vi "数据表比对.vi"(8 "error in (no error)":errorcluster, 9 "查询元素输入":string(combo), 10 "仪器日志参数":string, 11 "table输入":string(combo)) -> (0 "error out":errorcluster, 2 "待发送第一条数据":string[](array[string]), 3 "待发送数据":string[][](table))   [LabVIEW 2016, in "数据传输系统.lvlib"]
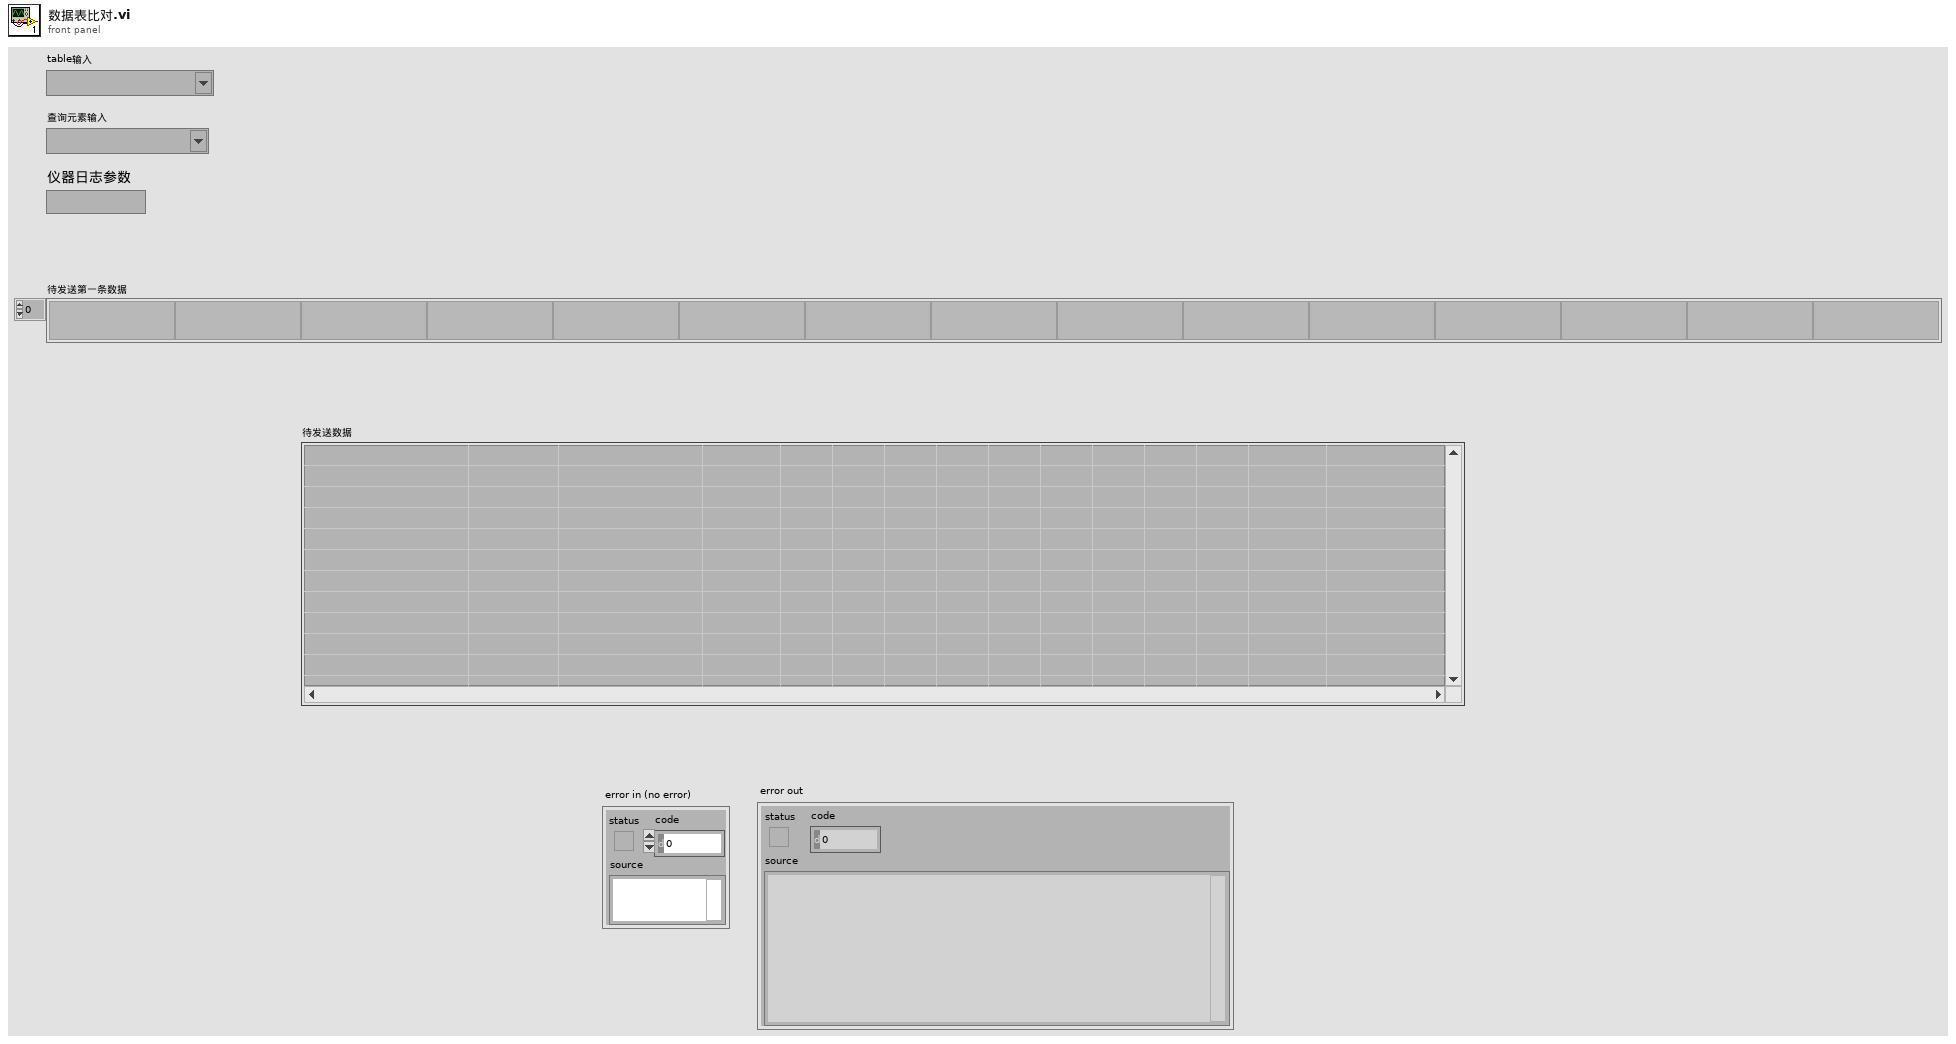
[diagram p1: front panel]
types:
  T1 = typedef "LVDateTimeRec.ctl" = cluster{"秒数的小数部分":dbl, "秒":i32, "分":i32, "时":i32, "日":i32, "月":i32, "年":i32, "天数（周）":i32, "天数（年）":i32, "DST":i32}
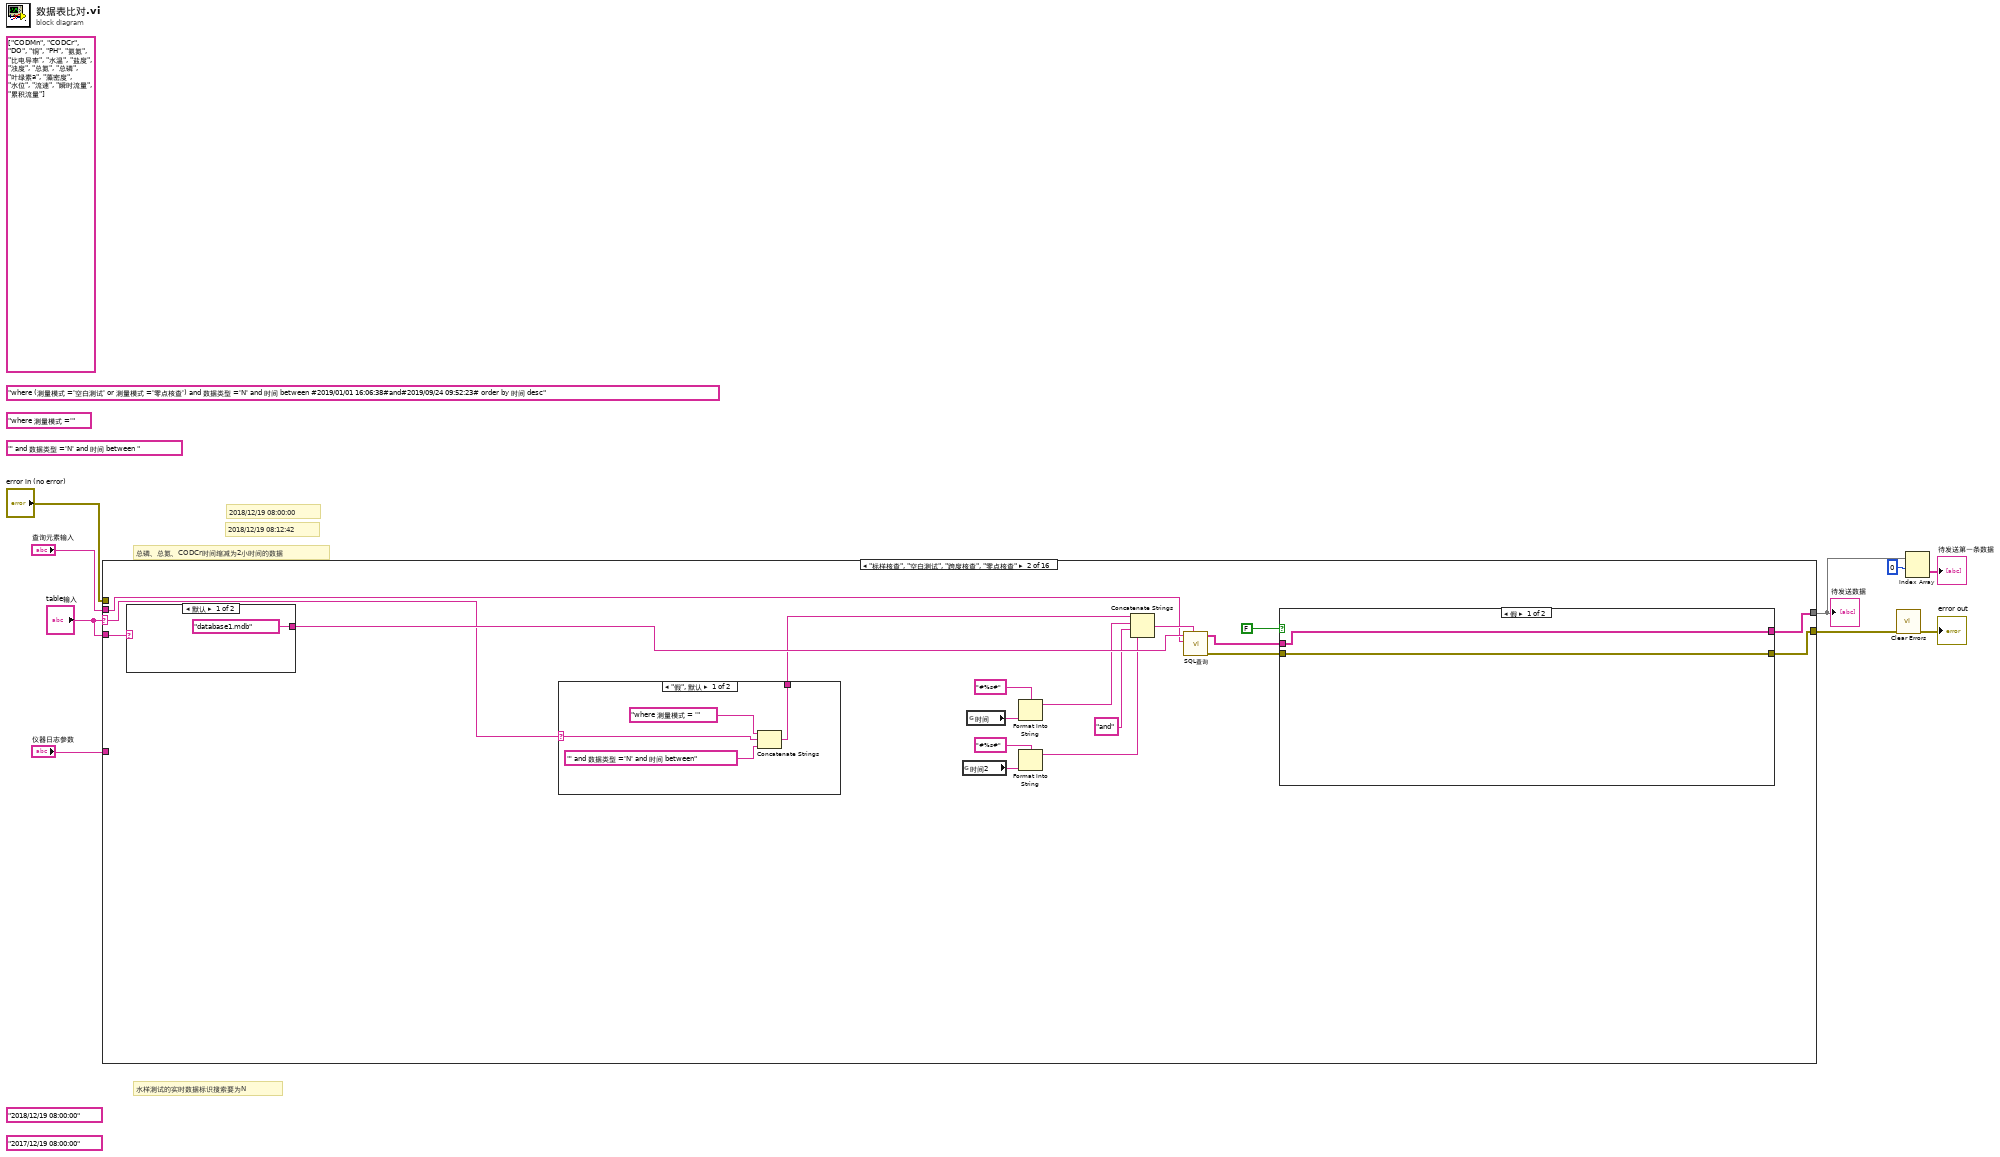
[diagram p0: block diagram]
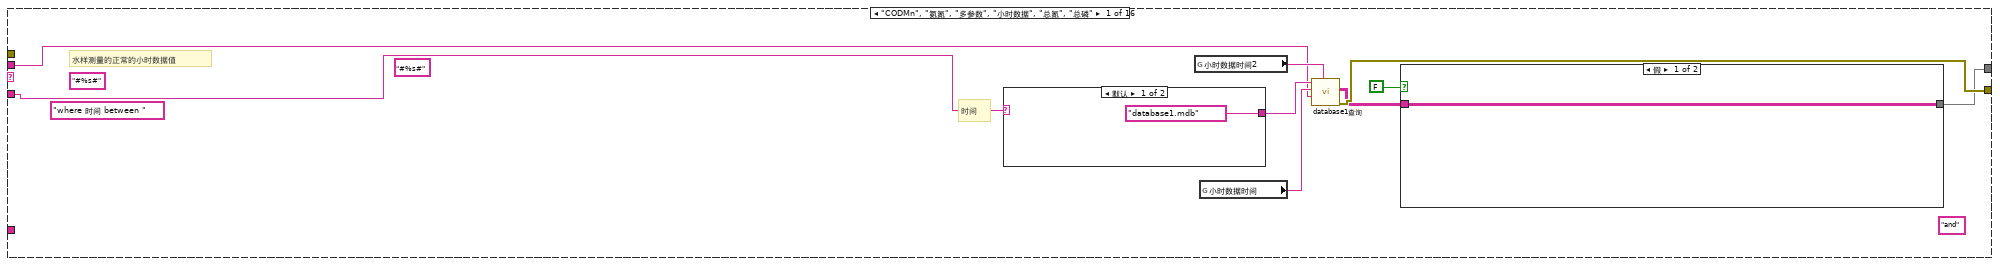
[diagram p2: hidden frame]
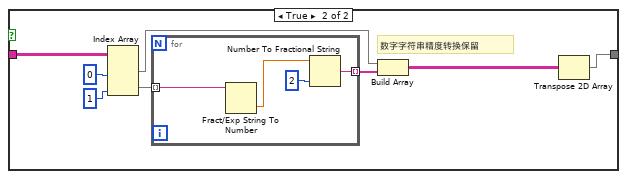
[diagram p3: hidden frame]
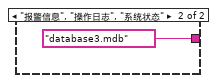
[diagram p4: hidden frame]
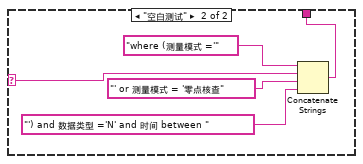
[diagram p5: hidden frame]
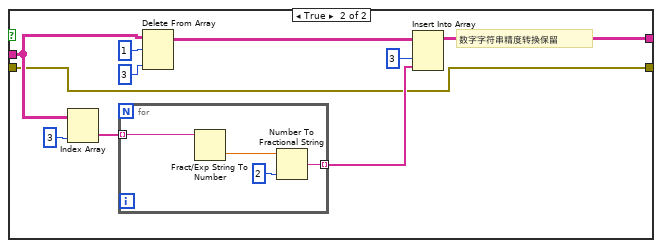
[diagram p6: hidden frame]
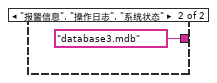
[diagram p7: hidden frame]
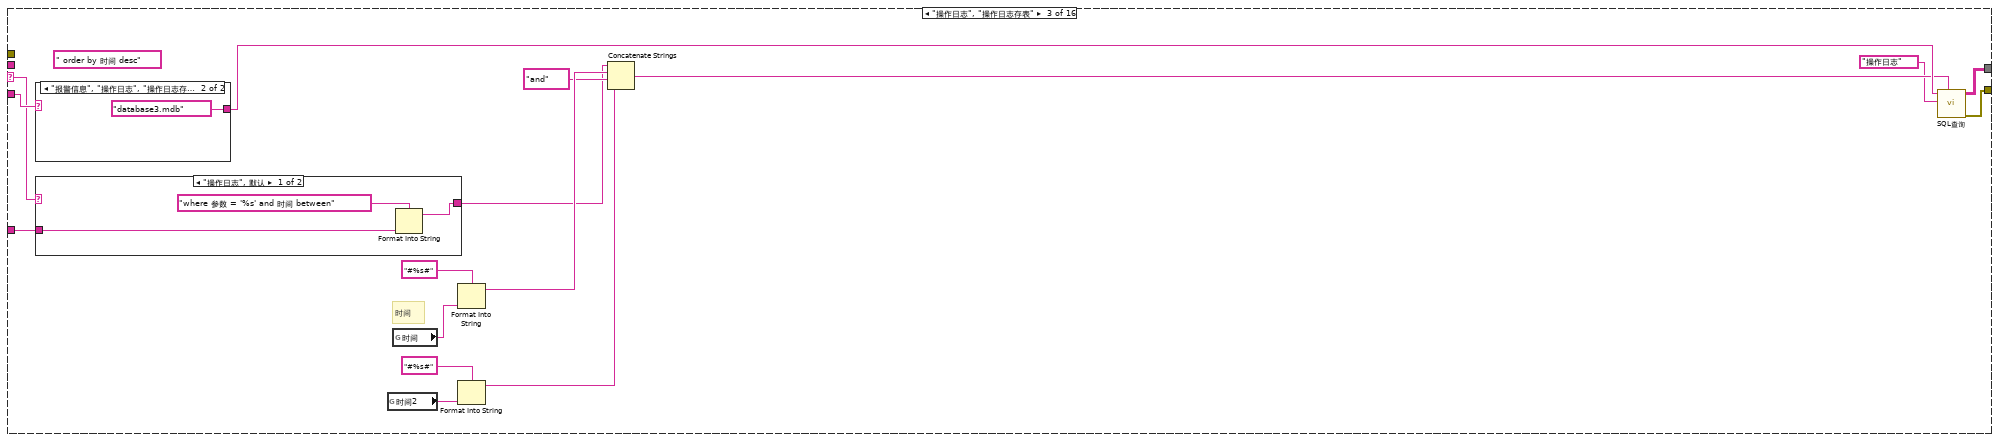
[diagram p8: hidden frame]
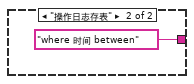
[diagram p9: hidden frame]
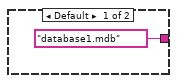
[diagram p10: hidden frame]
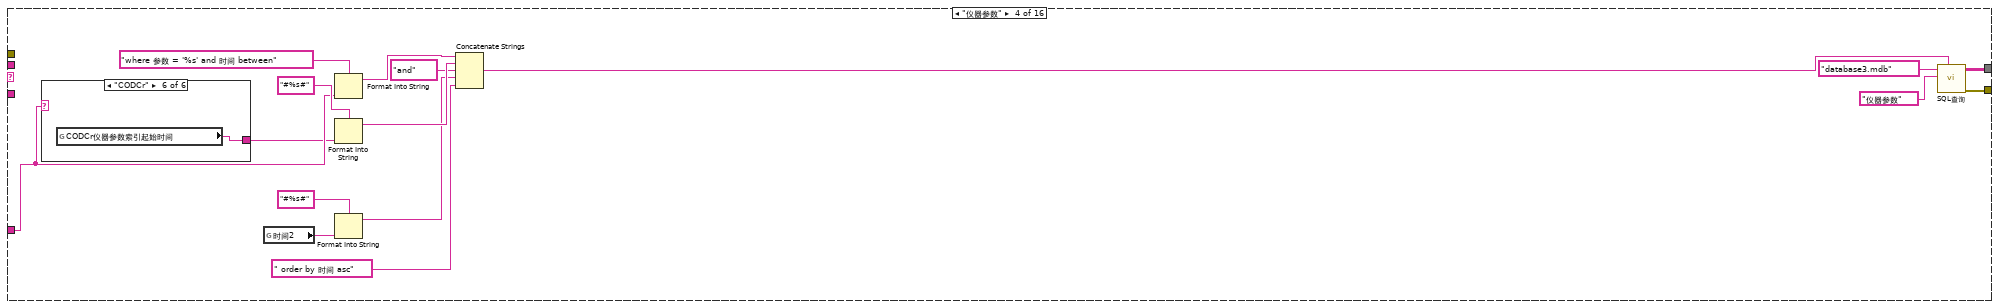
[diagram p11: hidden frame]
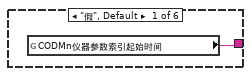
[diagram p12: hidden frame]
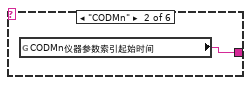
[diagram p13: hidden frame]
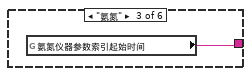
[diagram p14: hidden frame]
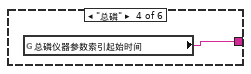
[diagram p15: hidden frame]
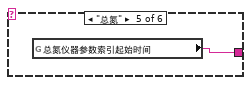
[diagram p16: hidden frame]
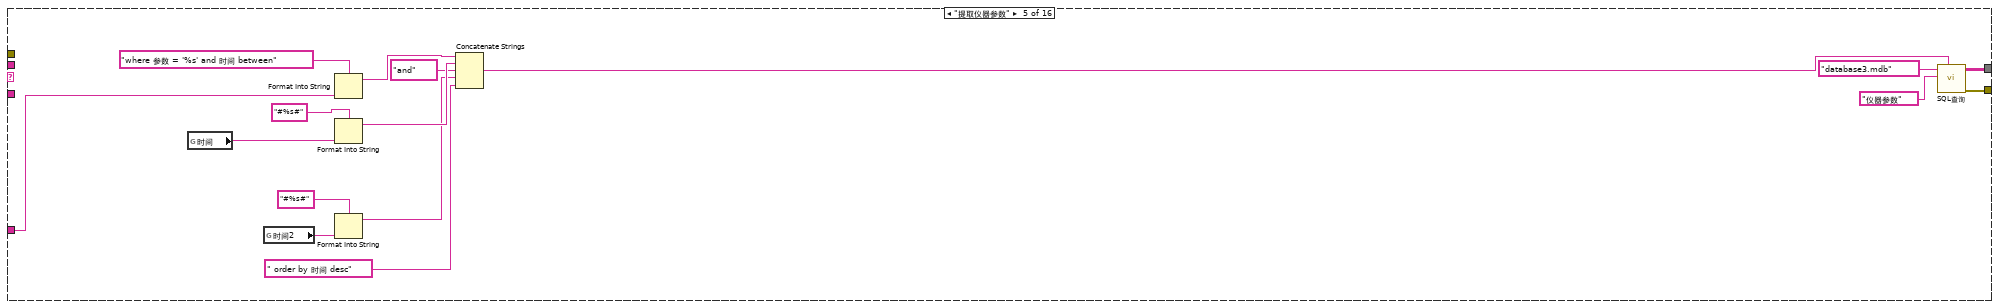
[diagram p17: hidden frame]
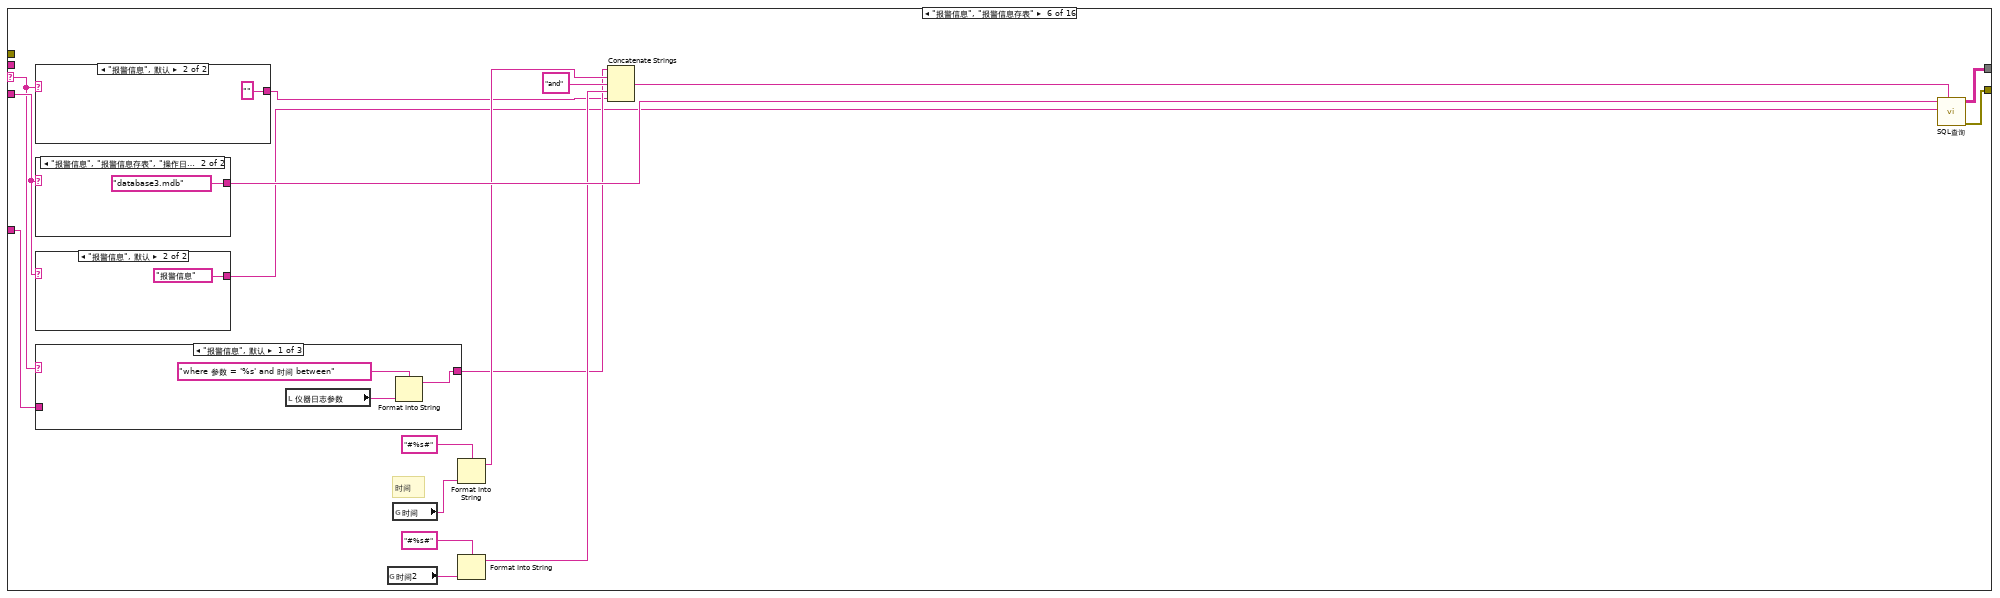
[diagram p18: hidden frame]
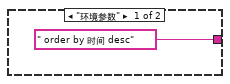
[diagram p19: hidden frame]
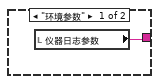
[diagram p20: hidden frame]
diagram:
  (unwired) "' and 数据类型 ='N' and 时间 between "
  (unwired) "where 测量模式 ='" ("condition")
  (unwired) "where (测量模式 ='空白测试' or 测量模式 ='零点核查') and 数据类型 ='N' and 时间 between #2019/01/01 16:06:38#and#2019/09/24 09:52:23# order by 时间 desc" ("condition")
  (unwired) string[] ["CODMn", "CODCr", "DO", "铜", "PH", "氨氮", "比电导率", "水温", "盐度", "浊度", "总氮", "总磷", "叶绿素a", "藻密度", "水位", "流速", "瞬时流量", "累积流量"] ("查询参数数组")
  (unwired) "2017/12/19 08:00:00"
  (unwired) "2018/12/19 08:00:00"
  # "水样测试的实时数据标识搜索要为N"
  # "2018/12/19 08:00:00"
  # "总磷、总氮、CODCr时间缩减为2小时间的数据"
  # "2018/12/19 08:12:42"
  n1 = case shown="\"标样核查\", \"空白测试\", \"跨度核查\", \"零点核查\"" "table输入" {
    selector: "table输入" -> [_ w35 w80 _ _ w139 _ _ _ _ _ _ _ _ _ _]
    tunnel: "error in (no error)" -> [_ _ _ _ _ _ _ w200 _ _ _ _ _ _ _ _]
    tunnel: [w16 w37 w92 w115 w137 w154 w187 w200 w215 w312 w357 w409 w461 w501 w541 w579] -> w7
    tunnel: [w12 w40 w90 w113 w135 w152 w185 w198 w218 w315 w360 w412 w464 w504 w544 w581] -> w3
    tunnel: "table输入" -> [w18 w51 w94 _ _ w142 w177 _ _ _ _ _ _ _ _ _]
    tunnel: "查询元素输入" -> [w10 w36 _ _ _ _ _ _ w201 w301 w346 w398 w454 w494 w534 w574]
    tunnel: "仪器日志参数" -> [_ _ w79 w102 w124 w140 w169 _ _ _ _ _ _ _ _ _]
    frame "CODMn", "氨氮", "多参数", "小时数据", "总氮", "总磷" {
      (unwired) "and" ("字符串")
      (unwired) "#%s#" ("初始字符串")
      (unwired) "#%s#" ("初始字符串")
      (unwired) "where 时间 between " ("condition")
      # "水样测量的正常的小时数据值"
      # "时间"
      n2 = case shown="默认" w18 {
        tunnel: ["database1.mdb" ("database") "database3.mdb" ("database")] -> w17
        frame Default {
        }
        frame "报警信息", "操作日志", "系统状态" {
        }
      }
      n3 = global read "全局 时间2.vi" "小时数据时间2"() -> (w14:string)
      n4 = global read "全局 水样时间.vi" "小时数据时间"() -> (w15:string)
      n5 = call "database1查询.vi"("时间2"=w14, "table"=w10, "时间1"=w15, "database"=w17) -> ("error out"=w16:errorcluster, "data"=w13:string[][])  [unwired: 4 in, 1 out]
      n6 = case shown="假" FALSE {
        tunnel: w13 -> [w19 w27]
        tunnel: [w19 w20] -> w12
        frame False {
        }
        frame True {
          # "数字字符串精度转换保留"
          n7 = Index Array(array=w27, index (col) #1=0 ("禁用的索引 (列)"), index (col) #2=1 ("索引 (列)")) -> (element #1=w23:string[], element #2=w24:string[])  [unwired: 2 in]
          n8 = for {
            tunnel: w24 -> [w29] mode=indexing
            tunnel: [w28] -> w22 mode=indexing
            n9 = Fract/Exp String To Number(string=w29) -> (number=w30:dbl)  [unwired: 3 in, 1 out]
            n10 = Number To Fractional String(number=w30, precision (6)=i16 2 ("精度(6)")) -> (F-format string=w28:string)  [unwired: 2 in]
          }
          n11 = Build Array(w23, w22) -> (w21:string[][])
          n12 = Transpose 2D Array(2D array=w21) -> (transposed array=w20:string[][])
        }
      }
    }
    frame "标样核查", "空白测试", "跨度核查", "零点核查" {
      n13 = case shown="默认" w51 {
        tunnel: ["database1.mdb" ("database") "database3.mdb" ("database")] -> w50
        frame Default {
        }
        frame "报警信息", "操作日志", "系统状态" {
        }
      }
      n14 = case shown="\"假\", 默认" w35 {
        selector: w35 -> [w54 w57]
        tunnel: [w52 w56] -> w34
        frame "假", Default {
          n15 = Concatenate Strings("where 测量模式 = '" ("condition"), w54, "' and 数据类型 ='N' and 时间 between" ("字符串")) -> (w52:string)
        }
        frame "空白测试" {
          n16 = Concatenate Strings("where (测量模式 ='" ("condition"), w57, "' or 测量模式 = '零点核查", "') and 数据类型 ='N' and 时间 between ") -> (w56:string)
        }
      }
      n17 = global read "全局 时间2.vi" "时间2"() -> (w42:string)
      n18 = global read "全局 水样时间.vi" "时间"() -> (w43:string)
      n19 = Format Into String(format string="#%s#" ("初始字符串"), w43) -> (resulting string=w49:string)  [unwired: 2 in, 1 out]
      n20 = Format Into String(format string="#%s#" ("初始字符串"), w42) -> (resulting string=w45:string)  [unwired: 2 in, 1 out]
      n21 = Concatenate Strings(w34, w49, "and" ("字符串"), w45) -> (w44:string)
      n22 = call "SQL查询.vi"("condition"=w44, "table输入"=w36, "database"=w50) -> ("error out"=w38:errorcluster, "data"=w41:string[][])  [unwired: 7 in]
      n23 = case shown="假" FALSE {
        tunnel: w41 -> [w62 w65]
        tunnel: [w62 w64] -> w40
        tunnel: [w61 w63] -> w37
        tunnel: w38 -> [w61 w63]
        frame False {
        }
        frame True {
          # "数字字符串精度转换保留"
          n24 = Index Array(array=w65, index (col)=3 ("禁用的索引 (列)")) -> (element=w71:string[])  [unwired: 1 in]
          n25 = for {
            tunnel: w71 -> [w74] mode=indexing
            tunnel: [w73] -> w67 mode=indexing
            n26 = Fract/Exp String To Number(string=w74) -> (number=w75:dbl)  [unwired: 3 in, 1 out]
            n27 = Number To Fractional String(number=w75, precision (6)=i16 2 ("精度(6)")) -> (F-format string=w73:string)  [unwired: 2 in]
          }
          n28 = Delete From Array(array=w65, length=1 ("长度"), index (col)=3 ("禁用的索引 (列)")) -> (array with subset deleted=w68:string[][])  [unwired: 1 in, 1 out]
          n29 = Insert Into Array(array=w68, index (col)=3 ("禁用的索引 (列)"), new element=w67) -> (w64:string[][])  [unwired: 1 in]
        }
      }
    }
    frame "操作日志", "操作日志存表" {
      (unwired) " order by 时间 desc" ("字符串")
      # "时间"
      n30 = case shown="\"报警信息\", \"操作日志\", \"操作日志存表\", \"系统状态\"" w94 {
        tunnel: ["database1.mdb" ("database") "database3.mdb" ("database")] -> w93
        frame Default {
        }
        frame "报警信息", "操作日志", "操作日志存表", "系统状态" {
        }
      }
      n31 = case shown="\"操作日志\", 默认" w80 {
        tunnel: [w96 "where 时间 between" ("condition")] -> w82
        tunnel: w79 -> [w95 _]
        frame "操作日志", Default {
          n32 = Format Into String(format string="where 参数 = '%s' and 时间 between" ("condition"), w95) -> (resulting string=w96:string)  [unwired: 2 in, 1 out]
        }
        frame "操作日志存表" {
        }
      }
      n33 = global read "全局 时间2.vi" "时间2"() -> (w83:string)
      n34 = global read "全局 水样时间.vi" "时间"() -> (w84:string)
      n35 = Format Into String(format string="#%s#" ("初始字符串"), w84) -> (resulting string=w89:string)  [unwired: 2 in, 1 out]
      n36 = Format Into String(format string="#%s#" ("初始字符串"), w83) -> (resulting string=w85:string)  [unwired: 2 in, 1 out]
      n37 = Concatenate Strings(w82, w89, "and" ("字符串"), w85) -> (w91:string)
      n38 = call "SQL查询.vi"("condition"=w91, "table输入"="操作日志", "database"=w93) -> ("error out"=w92:errorcluster, "data"=w90:string[][])  [unwired: 7 in]
    }
    frame "仪器参数" {
      n39 = case shown="\"CODCr\"" w102 {
        tunnel: [w117 w118 w119 w120 w121 w122] -> w101
        frame "假", Default {
          n40 = global read "全局 时间2.vi" "CODMn仪器参数索引起始时间"() -> (w117:string)
        }
        frame "CODMn" {
          n41 = global read "全局 时间2.vi" "CODMn仪器参数索引起始时间"() -> (w118:string)
        }
        frame "氨氮" {
          n42 = global read "全局 时间2.vi" "氨氮仪器参数索引起始时间"() -> (w119:string)
        }
        frame "总磷" {
          n43 = global read "全局 时间2.vi" "总磷仪器参数索引起始时间"() -> (w120:string)
        }
        frame "总氮" {
          n44 = global read "全局 时间2.vi" "总氮仪器参数索引起始时间"() -> (w121:string)
        }
        frame "CODCr" {
          n45 = global read "全局 时间2.vi" "CODCr仪器参数索引起始时间"() -> (w122:string)
        }
      }
      n46 = global read "全局 时间2.vi" "时间2"() -> (w107:string)
      n47 = Format Into String(format string="where 参数 = '%s' and 时间 between" ("condition"), w102) -> (resulting string=w106:string)  [unwired: 2 in, 1 out]
      n48 = Format Into String(format string="#%s#" ("初始字符串"), w101) -> (resulting string=w112:string)  [unwired: 2 in, 1 out]
      n49 = Format Into String(format string="#%s#" ("初始字符串"), w107) -> (resulting string=w108:string)  [unwired: 2 in, 1 out]
      n50 = Concatenate Strings(w106, w112, "and" ("字符串"), w108, " order by 时间 asc" ("字符串")) -> (w114:string)
      n51 = call "SQL查询.vi"("condition"=w114, "table输入"="仪器参数", "database"="database3.mdb") -> ("error out"=w115:errorcluster, "data"=w113:string[][])  [unwired: 7 in]
    }
    frame "提取仪器参数" {
      n52 = global read "全局 水样时间.vi" "时间"() -> (w123:string)
      n53 = global read "全局 时间2.vi" "时间2"() -> (w129:string)
      n54 = Format Into String(format string="where 参数 = '%s' and 时间 between" ("condition"), w124) -> (resulting string=w128:string)  [unwired: 2 in, 1 out]
      n55 = Format Into String(format string="#%s#" ("初始字符串"), w123) -> (resulting string=w134:string)  [unwired: 2 in, 1 out]
      n56 = Format Into String(format string="#%s#" ("初始字符串"), w129) -> (resulting string=w130:string)  [unwired: 2 in, 1 out]
      n57 = Concatenate Strings(w128, w134, "and" ("字符串"), w130, " order by 时间 desc" ("字符串")) -> (w136:string)
      n58 = call "SQL查询.vi"("condition"=w136, "table输入"="仪器参数", "database"="database3.mdb") -> ("error out"=w137:errorcluster, "data"=w135:string[][])  [unwired: 7 in]
    }
    frame "报警信息", "报警信息存表" {
      # "时间"
      n59 = case shown="\"报警信息\", 默认" w139 {
        tunnel: [" order by 时间 desc" ("字符串") "" ("仪器日志参数")] -> w141
        frame "环境参数" {
        }
        frame "报警信息", Default {
        }
      }
      n60 = case shown="\"报警信息\", \"报警信息存表\", \"操作日志\", \"系统状态\"" w142 {
        tunnel: ["database1.mdb" ("database") "database3.mdb" ("database")] -> w155
        frame Default {
        }
        frame "报警信息", "报警信息存表", "操作日志", "系统状态" {
        }
      }
      n61 = case shown="\"报警信息\", 默认" w142 {
        tunnel: [w158 "报警信息" ("table输入")] -> w143
        frame "环境参数" {
          n62 = local read "仪器日志参数"() -> (w158:string)
        }
        frame "报警信息", Default {
        }
      }
      n63 = case shown="\"报警信息\", 默认" w139 {
        tunnel: [w161 w164 "where 时间 between" ("condition")] -> w144
        tunnel: w140 -> [_ w163 _]
        frame "报警信息", Default {
          n64 = local read "仪器日志参数"() -> (w160:string)
          n65 = Format Into String(format string="where 参数 = '%s' and 时间 between" ("condition"), w160) -> (resulting string=w161:string)  [unwired: 2 in, 1 out]
        }
        frame "环境参数" {
          n66 = Format Into String(format string="where 参数 = '%s' and 时间 between" ("condition"), w163) -> (resulting string=w164:string)  [unwired: 2 in, 1 out]
        }
        frame "报警信息存表" {
        }
      }
      n67 = global read "全局 时间2.vi" "时间2"() -> (w145:string)
      n68 = global read "全局 水样时间.vi" "时间"() -> (w146:string)
      n69 = Format Into String(format string="#%s#" ("初始字符串"), w146) -> (resulting string=w151:string)  [unwired: 2 in, 1 out]
      n70 = Format Into String(format string="#%s#" ("初始字符串"), w145) -> (resulting string=w147:string)  [unwired: 2 in, 1 out]
      n71 = Concatenate Strings(w144, w151, "and" ("字符串"), w147, w141) -> (w153:string)
      n72 = call "SQL查询.vi"("condition"=w153, "table输入"=w143, "database"=w155) -> ("error out"=w154:errorcluster, "data"=w152:string[][])  [unwired: 7 in]
    }
    frame "环境参数" {
      n73 = case shown="默认" w177 {
        tunnel: ["database1.mdb" ("database") "database3.mdb" ("database")] -> w188
        frame Default {
        }
        frame "报警信息", "报警信息存表", "操作日志", "系统状态" {
        }
      }
      n74 = case shown="\"环境参数\"" w169 {
        tunnel: [w192 "where 时间 between" ("condition") "where 时间 between" ("condition")] -> w179
        frame "报警信息", Default {
          n75 = local read "仪器日志参数"() -> (w191:string)
          n76 = Format Into String(format string="where 参数 = '%s' and 时间 between" ("condition"), w191) -> (resulting string=w192:string)  [unwired: 2 in, 1 out]
        }
        frame "环境参数" {
        }
        frame "报警信息存表" {
        }
      }
      n77 = case shown="\"环境参数\"" w177 {
        tunnel: [w189 "报警信息" ("table输入")] -> w178
        tunnel: w169 -> [w189 _]
        frame "环境参数" {
        }
        frame "报警信息", Default {
        }
      }
      n78 = Get Date/Time In Seconds() -> (seconds since 1Jan1904=w174:timestamp)
      n79 = Seconds To Date/Time(time stamp (now)=w174) -> (date time rec=w171:T1)  [unwired: 1 in]
      n80 = Date/Time To Seconds(2:w171) -> (0:w173:timestamp)  [unwired: 1 in]
      n81 = Format Date/Time String(time format string (%c)="%Y/%m/%d %H:%M:%S" ("时间格式字符串(%c)"), seconds (now)=w173) -> (date/time string=w170:string)  [unwired: 1 in]
      n82 = Format Into String(format string="#%s#" ("初始字符串"), w170) -> (resulting string=w180:string)  [unwired: 2 in, 1 out]
      n83 = Format Into String(format string="#%s#" ("初始字符串"), "1904/01/01 00:00:00") -> (resulting string=w184:string)  [unwired: 2 in, 1 out]
      n84 = Concatenate Strings(w179, w184, "and" ("字符串"), w180, " order by 时间 desc" ("字符串")) -> (w186:string)
      n85 = call "SQL查询.vi"("condition"=w186, "table输入"=w178, "database"=w188) -> ("error out"=w187:errorcluster, "data"=w185:string[][])  [unwired: 7 in]
    }
    frame Default {
      # "时间格式转换"
      n86 = local read "待发送数据"() -> (w199:string[][])
      n87 = call "数组时间戳格式化(子VI).vi"("待发送数据输入"=w199) -> ("待发送数据输出"=w198:string[][])  [unwired: 10 in]
    }
    frame "实时数据" {
      (unwired) " order by 时间 desc" ("字符串")
      # "空白测试or零点核查要加括号"
      # "上传本地时间点的实时数据"
      # "上传质控数据（空白测试，跨度核查，核查数据，平行样数据）"
      n88 = global read "全局 实时数据参数.vi" "实时数据参数"() -> (w211:string)
      n89 = case shown="\"空白测试\"" w211 {
        tunnel: [w235 w257 w268 w274] -> w212
        tunnel: w211 -> [w231 w256 _ w270]
        tunnel: [w234 w252 w264 w269] -> w206
        tunnel: w201 -> [_ w251 _ _]
        frame "水样测试" {
          n90 = Get Date/Time In Seconds() -> (seconds since 1Jan1904=w243:timestamp)
          n91 = Format Date/Time String(time format string (%c)="%Y%m%d%H%M%S%3u" ("时间格式字符串(%c)"), seconds (now)=w243) -> (date/time string=w241:string)  [unwired: 1 in]
          n92 = local read "查询元素输入"() -> (w236:string)
          n93 = Concatenate Strings("where 测量模式 ='" ("condition"), w231, "' and 数据类型 ='N' and 时间 between ") -> (w234:string)
          n94 = Replace Substring(2:8 ("长度（子字符串长度）"), 3:10 ("偏移量(0)"), 4:"0000" ("子字符串(\"\")"), 5:w241) -> (1:w237:string)  [unwired: 1 out]
          n95 = case shown="\"CODCr\", \"CODMn\", \"累积流量\", \"总氮\", \"总磷\"" w236 {
            tunnel: w237 -> [w245 w248 _]
            tunnel: [w244 w249 w250] -> w235
            frame Default {
              n96 = Search and Replace String(input string=w245, search string="." ("搜索字符串")) -> (result string=w246:string)  [unwired: 6 in, 3 out]
              n97 = call "格式时间字符串.vi"("字符串"=w246) -> ("连接的字符串"=w244:string)  [unwired: 10 in]
            }
            frame "CODCr", "CODMn", "累积流量", "总氮", "总磷" {
              n98 = call "实时数据查询用2小时间的数据.vi"("字符串"=w248) -> ("连接的字符串"=w249:string)  [unwired: 10 in]
            }
            frame "CODCr加标回收率", "CODMn加标回收率", "氨氮加标回收率", "总氮加标回收率", "总磷加标回收率" {
              n99 = global read "全局 时间2.vi" "加标回收索引起始时间"() -> (w250:string)
            }
          }
        }
        frame "空白测试" {
          n100 = case shown="\"氨氮\"" w251 {
            tunnel: [w258 w259 w260 w261 w262 w263] -> w257
            frame "CODMn" {
              n101 = global read "全局 时间2.vi" "CODMn零点核查索引起始时间"() -> (w258:string)
            }
            frame "CODCr" {
              n102 = global read "全局 时间2.vi" "CODCr零点核查索引起始时间"() -> (w259:string)
            }
            frame "氨氮" {
              n103 = global read "全局 时间2.vi" "氨氮零点核查索引起始时间"() -> (w260:string)
            }
            frame "总磷" {
              n104 = global read "全局 时间2.vi" "总磷零点核查索引起始时间"() -> (w261:string)
            }
            frame "总氮" {
              n105 = global read "全局 时间2.vi" "总氮零点核查索引起始时间"() -> (w262:string)
            }
            frame "", Default {
              n106 = global read "全局 时间2.vi" "零点核查索引起始时间"() -> (w263:string)
            }
          }
          n107 = Concatenate Strings("where (测量模式 ='" ("condition"), w256, "' or 测量模式 = '零点核查", "') and 数据类型 ='N' and 时间 between ") -> (w252:string)
        }
        frame "核查数据" {
          n108 = global read "全局 时间2.vi" "标样核查索引起始时间"() -> (w268:string)
          n109 = Concatenate Strings("where 测量模式 ='" ("condition"), "标样核查" ("实时数据参数"), "' and 数据类型 ='N' and 时间 between ") -> (w264:string)
        }
        frame "跨度核查", Default {
          n110 = local read "查询元素输入"() -> (w273:string)
          n111 = Concatenate Strings("where 测量模式 ='" ("condition"), w270, "' and 数据类型 ='N' and 时间 between ") -> (w269:string)
          n112 = case shown="\"氨氮\"" w273 {
            tunnel: [w275 w276 w277 w278 w279 w280] -> w274
            frame "CODMn" {
              n113 = global read "全局 时间2.vi" "CODMn跨度核查索引起始时间"() -> (w275:string)
            }
            frame "CODCr" {
              n114 = global read "全局 时间2.vi" "CODCr跨度核查索引起始时间"() -> (w276:string)
            }
            frame "氨氮" {
              n115 = global read "全局 时间2.vi" "氨氮跨度核查索引起始时间"() -> (w277:string)
            }
            frame "总磷" {
              n116 = global read "全局 时间2.vi" "总磷跨度核查索引起始时间"() -> (w278:string)
            }
            frame "总氮" {
              n117 = global read "全局 时间2.vi" "总氮跨度核查索引起始时间"() -> (w279:string)
            }
            frame "", Default {
              n118 = global read "全局 时间2.vi" "跨度核查索引起始时间"() -> (w280:string)
            }
          }
        }
      }
      n119 = global read "断电保存全局.vi" "数据组合发送"() -> (w203:bool)
      n120 = Get Date/Time In Seconds() -> (seconds since 1Jan1904=w210:timestamp)
      n121 = Seconds To Date/Time(time stamp (now)=w210) -> (date time rec=w205:T1)  [unwired: 1 in]
      n122 = case shown="假" w203 {
        tunnel: w205 -> [w225 w228]
        tunnel: [w225 w226] -> w204
        frame False {
        }
        frame True {
          n123 = Unbundle By Name(w228) -> ("时"=w230:i32)
          n124 = Subtract(x=w230, y=2) -> (x-y=w227:i32)
          n125 = Bundle By Name(cluster=w228, "时"=w227) -> (w226:T1)
        }
      }
      n126 = Date/Time To Seconds(2:w204) -> (0:w209:timestamp)  [unwired: 1 in]
      n127 = Format Date/Time String(time format string (%c)="%Y/%m/%d %H:%M:%S" ("时间格式字符串(%c)"), seconds (now)=w209) -> (date/time string=w207:string)  [unwired: 1 in]
      n128 = Format Into String(format string="#%s#" ("初始字符串"), w212) -> (resulting string=w224:string)  [unwired: 2 in, 1 out]
      n129 = Format Into String(format string="#%s#" ("初始字符串"), w207) -> (resulting string=w220:string)  [unwired: 2 in, 1 out]
      n130 = Concatenate Strings(w206, w224, "and" ("字符串"), w220, " order by 时间 asc" ("字符串")) -> (w214:string)
      n131 = call "SQL查询.vi"("condition"=w214, "table输入"=w201, "database"="database1.mdb") -> ("error out"=w216:errorcluster, "data"=w213:string[][])  [unwired: 7 in]
      n132 = case shown="\"CODCr\", \"总氮\", \"总磷\"" w201 {
        tunnel: w201 -> [_ w283]
        tunnel: w214 -> [_ w282]
        tunnel: w213 -> [_ w281]
        frame Default {
        }
        frame "CODCr", "总氮", "总磷" {
          n133 = global write "全局 实时数据参数.vi" "data"(w281) -> ()
          n134 = global write "全局 实时数据参数.vi" "参数"(w283) -> ()
          n135 = global write "全局 实时数据参数.vi" "连接的字符串"(w282) -> ()
        }
      }
      n136 = case shown="假" FALSE {
        tunnel: [w285 w288] -> w218
        tunnel: w213 -> [w285 w287]
        tunnel: w216 -> [w284 w286]
        tunnel: [w284 w286] -> w215
        frame False {
        }
        frame True {
          # "数字字符串精度转换保留"
          n137 = Index Array(array=w287, index (col)=3 ("禁用的索引 (列)")) -> (element=w294:string[])  [unwired: 1 in]
          n138 = for {
            tunnel: w294 -> [w297] mode=indexing
            tunnel: [w296] -> w290 mode=indexing
            n139 = Fract/Exp String To Number(string=w297) -> (number=w298:dbl)  [unwired: 3 in, 1 out]
            n140 = Number To Fractional String(number=w298, precision (6)=i16 2 ("精度(6)")) -> (F-format string=w296:string)  [unwired: 2 in]
          }
          n141 = Delete From Array(array=w287, length=1 ("长度"), index (col)=3 ("禁用的索引 (列)")) -> (array with subset deleted=w291:string[][])  [unwired: 1 in, 1 out]
          n142 = Insert Into Array(array=w291, index (col)=3 ("禁用的索引 (列)"), new element=w290) -> (w288:string[][])  [unwired: 1 in]
        }
      }
    }
    frame "加标回收" {
      w307 = "加标回收率" ("字符串")
      # "上传加标回收数据"
      n143 = global read "全局 数据发送重叠.vi" "掉线指示灯"() -> (w308:bool)
      n144 = case shown="假" w308 {
        tunnel: [w324 w325] -> w309
        frame False {
          n145 = global read "全局 时间2.vi" "加标回收索引起始时间"() -> (w324:string)
        }
        frame True {
          n146 = global read "全局 数据发送重叠.vi" "TCP掉线时间节点"() -> (w325:string)
        }
      }
      n147 = Get Date/Time In Seconds() -> (seconds since 1Jan1904=w306:timestamp)
      n148 = Seconds To Date/Time(time stamp (now)=w306) -> (date time rec=w303:T1)  [unwired: 1 in]
      n149 = Date/Time To Seconds(2:w303) -> (0:w305:timestamp)  [unwired: 1 in]
      n150 = Format Date/Time String(time format string (%c)="%Y/%m/%d %H:%M:%S" ("时间格式字符串(%c)"), seconds (now)=w305) -> (date/time string=w302:string)  [unwired: 1 in]
      n151 = Format Into String(format string="#%s#" ("初始字符串"), w309) -> (resulting string=w323:string)  [unwired: 2 in, 1 out]
      n152 = Format Into String(format string="#%s#" ("初始字符串"), w302) -> (resulting string=w319:string)  [unwired: 2 in, 1 out]
      n153 = Concatenate Strings("where 参数 ='" ("condition"), w301, "' and 时间 between ", w323, "and" ("字符串"), w319, " order by 时间 asc" ("字符串")) -> (w311:string)
      n154 = call "SQL查询.vi"("condition"=w311, "table输入"=w307, "database"="database1.mdb") -> ("error out"=w313:errorcluster, "data"=w310:string[][])  [unwired: 7 in]
      n155 = case shown="\"CODCr\", \"总氮\", \"总磷\"" w307 {
        tunnel: w307 -> [_ w328]
        tunnel: w311 -> [_ w327]
        tunnel: w310 -> [_ w326]
        frame Default {
        }
        frame "CODCr", "总氮", "总磷" {
          n156 = global write "全局 实时数据参数.vi" "data"(w326) -> ()
          n157 = global write "全局 实时数据参数.vi" "参数"(w328) -> ()
          n158 = global write "全局 实时数据参数.vi" "连接的字符串"(w327) -> ()
        }
      }
      n159 = case shown="假" FALSE {
        tunnel: [w330 w333] -> w315
        tunnel: w310 -> [w330 w332]
        tunnel: w313 -> [w329 w331]
        tunnel: [w329 w331] -> w312
        frame False {
        }
        frame True {
          # "数字字符串精度转换保留"
          n160 = Index Array(array=w332, index (col)=3 ("禁用的索引 (列)")) -> (element=w339:string[])  [unwired: 1 in]
          n161 = for {
            tunnel: w339 -> [w342] mode=indexing
            tunnel: [w341] -> w335 mode=indexing
            n162 = Fract/Exp String To Number(string=w342) -> (number=w343:dbl)  [unwired: 3 in, 1 out]
            n163 = Number To Fractional String(number=w343, precision (6)=i16 2 ("精度(6)")) -> (F-format string=w341:string)  [unwired: 2 in]
          }
          n164 = Delete From Array(array=w332, length=1 ("长度"), index (col)=3 ("禁用的索引 (列)")) -> (array with subset deleted=w336:string[][])  [unwired: 1 in, 1 out]
          n165 = Insert Into Array(array=w336, index (col)=3 ("禁用的索引 (列)"), new element=w335) -> (w333:string[][])  [unwired: 1 in]
        }
      }
    }
    frame "平行样测试" {
      w352 = "平行样测试" ("字符串")
      # "上传本地时间点的实时数据"
      # "上传平行样数据"
      n166 = global read "全局 数据发送重叠.vi" "掉线指示灯"() -> (w353:bool)
      n167 = case shown="假" w353 {
        tunnel: [w370 w377] -> w354
        frame False {
          n168 = local read "查询元素输入"() -> (w369:string)
          n169 = case shown="\"CODCr\"" w369 {
            tunnel: [w371 w372 w373 w374 w375 w376] -> w370
            frame "CODMn" {
              n170 = global read "全局 时间2.vi" "CODMn平行样索引起始时间"() -> (w371:string)
            }
            frame "CODCr" {
              n171 = global read "全局 时间2.vi" "CODCr平行样索引起始时间"() -> (w372:string)
            }
            frame "氨氮" {
              n172 = global read "全局 时间2.vi" "氨氮平行样索引起始时间"() -> (w373:string)
            }
            frame "总磷" {
              n173 = global read "全局 时间2.vi" "总磷平行样索引起始时间"() -> (w374:string)
            }
            frame "总氮" {
              n174 = global read "全局 时间2.vi" "总磷平行样索引起始时间"() -> (w375:string)
            }
            frame "", Default {
              n175 = global read "全局 时间2.vi" "平行样索引起始时间"() -> (w376:string)
            }
          }
        }
        frame True {
          n176 = global read "全局 数据发送重叠.vi" "TCP掉线时间节点"() -> (w377:string)
        }
      }
      n177 = Get Date/Time In Seconds() -> (seconds since 1Jan1904=w351:timestamp)
      n178 = Seconds To Date/Time(time stamp (now)=w351) -> (date time rec=w348:T1)  [unwired: 1 in]
      n179 = Date/Time To Seconds(2:w348) -> (0:w350:timestamp)  [unwired: 1 in]
      n180 = Format Date/Time String(time format string (%c)="%Y/%m/%d %H:%M:%S" ("时间格式字符串(%c)"), seconds (now)=w350) -> (date/time string=w347:string)  [unwired: 1 in]
      n181 = Format Into String(format string="#%s#" ("初始字符串"), w354) -> (resulting string=w368:string)  [unwired: 2 in, 1 out]
      n182 = Format Into String(format string="#%s#" ("初始字符串"), w347) -> (resulting string=w364:string)  [unwired: 2 in, 1 out]
      n183 = Concatenate Strings("where 参数 ='" ("condition"), w346, "' and 时间 between ", w368, "and" ("字符串"), w364, " order by 时间 asc" ("字符串")) -> (w356:string)
      n184 = call "SQL查询.vi"("condition"=w356, "table输入"=w352, "database"="database1.mdb") -> ("error out"=w358:errorcluster, "data"=w355:string[][])  [unwired: 7 in]
      n185 = case shown="默认" w352 {
        tunnel: w352 -> [_ w380]
        tunnel: w356 -> [_ w379]
        tunnel: w355 -> [_ w378]
        frame Default {
        }
        frame "CODCr", "总氮", "总磷" {
          n186 = global write "全局 实时数据参数.vi" "data"(w378) -> ()
          n187 = global write "全局 实时数据参数.vi" "参数"(w380) -> ()
          n188 = global write "全局 实时数据参数.vi" "连接的字符串"(w379) -> ()
        }
      }
      n189 = case shown="假" FALSE {
        tunnel: [w382 w385] -> w360
        tunnel: w355 -> [w382 w384]
        tunnel: w358 -> [w381 w383]
        tunnel: [w381 w383] -> w357
        frame False {
        }
        frame True {
          # "数字字符串精度转换保留"
          n190 = Index Array(array=w384, index (col)=3 ("禁用的索引 (列)")) -> (element=w391:string[])  [unwired: 1 in]
          n191 = for {
            tunnel: w391 -> [w394] mode=indexing
            tunnel: [w393] -> w387 mode=indexing
            n192 = Fract/Exp String To Number(string=w394) -> (number=w395:dbl)  [unwired: 3 in, 1 out]
            n193 = Number To Fractional String(number=w395, precision (6)=i16 2 ("精度(6)")) -> (F-format string=w393:string)  [unwired: 2 in]
          }
          n194 = Delete From Array(array=w384, length=1 ("长度"), index (col)=3 ("禁用的索引 (列)")) -> (array with subset deleted=w388:string[][])  [unwired: 1 in, 1 out]
          n195 = Insert Into Array(array=w388, index (col)=3 ("禁用的索引 (列)"), new element=w387) -> (w385:string[][])  [unwired: 1 in]
        }
      }
    }
    frame "集成干预测试" {
      w404 = "集成干预测试" ("字符串")
      # "上传本地时间点的实时数据"
      # "上传集成干预数据"
      n196 = global read "全局 数据发送重叠.vi" "掉线指示灯"() -> (w405:bool)
      n197 = case shown="假" w405 {
        tunnel: [w422 w434] -> w406
        frame False {
          n198 = local read "查询元素输入"() -> (w421:string)
          n199 = case shown="\"CODMn\"" w421 {
            tunnel: [w423 w424 w425 w426 w427 w428 w429 w430 w431 w432 w433] -> w422
            frame "CODMn" {
              n200 = global read "全局 时间2.vi" "CODMn集成干预索引起始时间"() -> (w423:string)
            }
            frame "CODCr" {
              n201 = global read "全局 时间2.vi" "CODCr集成干预索引起始时间"() -> (w424:string)
            }
            frame "氨氮" {
              n202 = global read "全局 时间2.vi" "氨氮集成干预索引起始时间"() -> (w425:string)
            }
            frame "总磷" {
              n203 = global read "全局 时间2.vi" "总磷集成干预索引起始时间"() -> (w426:string)
            }
            frame "总氮" {
              n204 = global read "全局 时间2.vi" "总氮集成干预索引起始时间"() -> (w427:string)
            }
            frame "DO" {
              n205 = global read "全局 时间2.vi" "DO集成干预索引起始时间"() -> (w428:string)
            }
            frame "PH" {
              n206 = global read "全局 时间2.vi" "PH集成干预索引起始时间"() -> (w429:string)
            }
            frame "比电导率" {
              n207 = global read "全局 时间2.vi" "比电导率集成干预索引起始时间"() -> (w430:string)
            }
            frame "水温" {
              n208 = global read "全局 时间2.vi" "水温集成干预索引起始时间"() -> (w431:string)
            }
            frame "浊度" {
              n209 = global read "全局 时间2.vi" "浊度集成干预索引起始时间"() -> (w432:string)
            }
            frame "", Default {
              n210 = global read "全局 时间2.vi" "平行样索引起始时间"() -> (w433:string)
            }
          }
        }
        frame True {
          n211 = global read "全局 数据发送重叠.vi" "TCP掉线时间节点"() -> (w434:string)
        }
      }
      n212 = Get Date/Time In Seconds() -> (seconds since 1Jan1904=w403:timestamp)
      n213 = Seconds To Date/Time(time stamp (now)=w403) -> (date time rec=w400:T1)  [unwired: 1 in]
      n214 = Date/Time To Seconds(2:w400) -> (0:w402:timestamp)  [unwired: 1 in]
      n215 = Format Date/Time String(time format string (%c)="%Y/%m/%d %H:%M:%S" ("时间格式字符串(%c)"), seconds (now)=w402) -> (date/time string=w399:string)  [unwired: 1 in]
      n216 = Format Into String(format string="#%s#" ("初始字符串"), w406) -> (resulting string=w420:string)  [unwired: 2 in, 1 out]
      n217 = Format Into String(format string="#%s#" ("初始字符串"), w399) -> (resulting string=w416:string)  [unwired: 2 in, 1 out]
      n218 = Concatenate Strings("where 参数 ='" ("condition"), w398, "' and 时间 between ", w420, "and" ("字符串"), w416, " order by 时间 asc" ("字符串")) -> (w408:string)
      n219 = call "SQL查询.vi"("condition"=w408, "table输入"=w404, "database"="database1.mdb") -> ("error out"=w410:errorcluster, "data"=w407:string[][])  [unwired: 7 in]
      n220 = case shown="\"CODCr\", \"总氮\", \"总磷\"" w404 {
        tunnel: w404 -> [_ w437]
        tunnel: w408 -> [_ w436]
        tunnel: w407 -> [_ w435]
        frame Default {
        }
        frame "CODCr", "总氮", "总磷" {
          n221 = global write "全局 实时数据参数.vi" "data"(w435) -> ()
          n222 = global write "全局 实时数据参数.vi" "参数"(w437) -> ()
          n223 = global write "全局 实时数据参数.vi" "连接的字符串"(w436) -> ()
        }
      }
      n224 = case shown="假" FALSE {
        tunnel: [w439 w442] -> w412
        tunnel: w407 -> [w439 w441]
        tunnel: w410 -> [w438 w440]
        tunnel: [w438 w440] -> w409
        frame False {
        }
        frame True {
          # "数字字符串精度转换保留"
          n225 = Index Array(array=w441, index (col)=3 ("禁用的索引 (列)")) -> (element=w448:string[])  [unwired: 1 in]
          n226 = for {
            tunnel: w448 -> [w451] mode=indexing
            tunnel: [w450] -> w444 mode=indexing
            n227 = Fract/Exp String To Number(string=w451) -> (number=w452:dbl)  [unwired: 3 in, 1 out]
            n228 = Number To Fractional String(number=w452, precision (6)=i16 2 ("精度(6)")) -> (F-format string=w450:string)  [unwired: 2 in]
          }
          n229 = Delete From Array(array=w441, length=1 ("长度"), index (col)=3 ("禁用的索引 (列)")) -> (array with subset deleted=w445:string[][])  [unwired: 1 in, 1 out]
          n230 = Insert Into Array(array=w445, index (col)=3 ("禁用的索引 (列)"), new element=w444) -> (w442:string[][])  [unwired: 1 in]
        }
      }
    }
    frame "提取加标回收" {
      w456 = "加标回收率" ("字符串")
      # "上传本地时间点的实时数据"
      n231 = global read "全局 数据发送重叠.vi" "掉线指示灯"() -> (w457:bool)
      n232 = case shown="假" w457 {
        tunnel: [w473 w474] -> w458
        frame False {
          n233 = global read "起始时间.vi" "起始时间"() -> (w473:string)
        }
        frame True {
          n234 = global read "全局 数据发送重叠.vi" "TCP掉线时间节点"() -> (w474:string)
        }
      }
      n235 = global read "起始时间.vi" "结束时间"() -> (w455:string)
      n236 = Format Into String(format string="#%s#" ("初始字符串"), w458) -> (resulting string=w472:string)  [unwired: 2 in, 1 out]
      n237 = Format Into String(format string="#%s#" ("初始字符串"), w455) -> (resulting string=w468:string)  [unwired: 2 in, 1 out]
      n238 = Concatenate Strings("where 参数 ='" ("condition"), w454, "' and 时间 between ", w472, "and" ("字符串"), w468) -> (w460:string)
      n239 = call "SQL查询.vi"("condition"=w460, "table输入"=w456, "database"="database1.mdb") -> ("error out"=w462:errorcluster, "data"=w459:string[][])  [unwired: 7 in]
      n240 = case shown="\"CODCr\", \"总氮\", \"总磷\"" w456 {
        tunnel: w456 -> [_ w477]
        tunnel: w460 -> [_ w476]
        tunnel: w459 -> [_ w475]
        frame Default {
        }
        frame "CODCr", "总氮", "总磷" {
          n241 = global write "全局 实时数据参数.vi" "data"(w475) -> ()
          n242 = global write "全局 实时数据参数.vi" "参数"(w477) -> ()
          n243 = global write "全局 实时数据参数.vi" "连接的字符串"(w476) -> ()
        }
      }
      n244 = case shown="假" FALSE {
        tunnel: [w479 w482] -> w464
        tunnel: w459 -> [w479 w481]
        tunnel: w462 -> [w478 w480]
        tunnel: [w478 w480] -> w461
        frame False {
        }
        frame True {
          # "数字字符串精度转换保留"
          n245 = Index Array(array=w481, index (col)=3 ("禁用的索引 (列)")) -> (element=w488:string[])  [unwired: 1 in]
          n246 = for {
            tunnel: w488 -> [w491] mode=indexing
            tunnel: [w490] -> w484 mode=indexing
            n247 = Fract/Exp String To Number(string=w491) -> (number=w492:dbl)  [unwired: 3 in, 1 out]
            n248 = Number To Fractional String(number=w492, precision (6)=i16 2 ("精度(6)")) -> (F-format string=w490:string)  [unwired: 2 in]
          }
          n249 = Delete From Array(array=w481, length=1 ("长度"), index (col)=3 ("禁用的索引 (列)")) -> (array with subset deleted=w485:string[][])  [unwired: 1 in, 1 out]
          n250 = Insert Into Array(array=w485, index (col)=3 ("禁用的索引 (列)"), new element=w484) -> (w482:string[][])  [unwired: 1 in]
        }
      }
    }
    frame "提取平行样" {
      w496 = "平行样测试" ("字符串")
      # "上传本地时间点的实时数据"
      n251 = global read "全局 数据发送重叠.vi" "掉线指示灯"() -> (w497:bool)
      n252 = case shown="假" w497 {
        tunnel: [w513 w514] -> w498
        frame False {
          n253 = global read "起始时间.vi" "起始时间"() -> (w513:string)
        }
        frame True {
          n254 = global read "全局 数据发送重叠.vi" "TCP掉线时间节点"() -> (w514:string)
        }
      }
      n255 = global read "起始时间.vi" "结束时间"() -> (w495:string)
      n256 = Format Into String(format string="#%s#" ("初始字符串"), w498) -> (resulting string=w512:string)  [unwired: 2 in, 1 out]
      n257 = Format Into String(format string="#%s#" ("初始字符串"), w495) -> (resulting string=w508:string)  [unwired: 2 in, 1 out]
      n258 = Concatenate Strings("where 参数 ='" ("condition"), w494, "' and 时间 between ", w512, "and" ("字符串"), w508) -> (w500:string)
      n259 = call "SQL查询.vi"("condition"=w500, "table输入"=w496, "database"="database1.mdb") -> ("error out"=w502:errorcluster, "data"=w499:string[][])  [unwired: 7 in]
      n260 = case shown="\"CODCr\", \"总氮\", \"总磷\"" w496 {
        tunnel: w496 -> [_ w517]
        tunnel: w500 -> [_ w516]
        tunnel: w499 -> [_ w515]
        frame Default {
        }
        frame "CODCr", "总氮", "总磷" {
          n261 = global write "全局 实时数据参数.vi" "data"(w515) -> ()
          n262 = global write "全局 实时数据参数.vi" "参数"(w517) -> ()
          n263 = global write "全局 实时数据参数.vi" "连接的字符串"(w516) -> ()
        }
      }
      n264 = case shown="假" FALSE {
        tunnel: [w519 w522] -> w504
        tunnel: w499 -> [w519 w521]
        tunnel: w502 -> [w518 w520]
        tunnel: [w518 w520] -> w501
        frame False {
        }
        frame True {
          # "数字字符串精度转换保留"
          n265 = Index Array(array=w521, index (col)=3 ("禁用的索引 (列)")) -> (element=w528:string[])  [unwired: 1 in]
          n266 = for {
            tunnel: w528 -> [w531] mode=indexing
            tunnel: [w530] -> w524 mode=indexing
            n267 = Fract/Exp String To Number(string=w531) -> (number=w532:dbl)  [unwired: 3 in, 1 out]
            n268 = Number To Fractional String(number=w532, precision (6)=i16 2 ("精度(6)")) -> (F-format string=w530:string)  [unwired: 2 in]
          }
          n269 = Delete From Array(array=w521, length=1 ("长度"), index (col)=3 ("禁用的索引 (列)")) -> (array with subset deleted=w525:string[][])  [unwired: 1 in, 1 out]
          n270 = Insert Into Array(array=w525, index (col)=3 ("禁用的索引 (列)"), new element=w524) -> (w522:string[][])  [unwired: 1 in]
        }
      }
    }
    frame "提取集成干预" {
      w536 = "集成干预测试" ("字符串")
      # "上传本地时间点的实时数据"
      n271 = global read "全局 数据发送重叠.vi" "掉线指示灯"() -> (w537:bool)
      n272 = case shown="假" w537 {
        tunnel: [w553 w554] -> w538
        frame False {
          n273 = global read "起始时间.vi" "起始时间"() -> (w553:string)
        }
        frame True {
          n274 = global read "全局 数据发送重叠.vi" "TCP掉线时间节点"() -> (w554:string)
        }
      }
      n275 = global read "起始时间.vi" "结束时间"() -> (w535:string)
      n276 = Format Into String(format string="#%s#" ("初始字符串"), w538) -> (resulting string=w552:string)  [unwired: 2 in, 1 out]
      n277 = Format Into String(format string="#%s#" ("初始字符串"), w535) -> (resulting string=w548:string)  [unwired: 2 in, 1 out]
      n278 = Concatenate Strings("where 参数 ='" ("condition"), w534, "' and 时间 between ", w552, "and" ("字符串"), w548) -> (w540:string)
      n279 = call "SQL查询.vi"("condition"=w540, "table输入"=w536, "database"="database1.mdb") -> ("error out"=w542:errorcluster, "data"=w539:string[][])  [unwired: 7 in]
      n280 = case shown="\"CODCr\", \"总氮\", \"总磷\"" w536 {
        tunnel: w536 -> [_ w557]
        tunnel: w540 -> [_ w556]
        tunnel: w539 -> [_ w555]
        frame Default {
        }
        frame "CODCr", "总氮", "总磷" {
          n281 = global write "全局 实时数据参数.vi" "data"(w555) -> ()
          n282 = global write "全局 实时数据参数.vi" "参数"(w557) -> ()
          n283 = global write "全局 实时数据参数.vi" "连接的字符串"(w556) -> ()
        }
      }
      n284 = case shown="假" FALSE {
        tunnel: [w559 w562] -> w544
        tunnel: w539 -> [w559 w561]
        tunnel: w542 -> [w558 w560]
        tunnel: [w558 w560] -> w541
        frame False {
        }
        frame True {
          # "数字字符串精度转换保留"
          n285 = Index Array(array=w561, index (col)=3 ("禁用的索引 (列)")) -> (element=w568:string[])  [unwired: 1 in]
          n286 = for {
            tunnel: w568 -> [w571] mode=indexing
            tunnel: [w570] -> w564 mode=indexing
            n287 = Fract/Exp String To Number(string=w571) -> (number=w572:dbl)  [unwired: 3 in, 1 out]
            n288 = Number To Fractional String(number=w572, precision (6)=i16 2 ("精度(6)")) -> (F-format string=w570:string)  [unwired: 2 in]
          }
          n289 = Delete From Array(array=w561, length=1 ("长度"), index (col)=3 ("禁用的索引 (列)")) -> (array with subset deleted=w565:string[][])  [unwired: 1 in, 1 out]
          n290 = Insert Into Array(array=w565, index (col)=3 ("禁用的索引 (列)"), new element=w564) -> (w562:string[][])  [unwired: 1 in]
        }
      }
    }
    frame "提取实时数据" {
      # "上传给定时间段之间的实时数据"
      n291 = global read "起始时间.vi" "起始时间"() -> (w584:string)
      n292 = global read "起始时间.vi" "结束时间"() -> (w583:string)
      n293 = global read "全局 实时数据参数.vi" "实时数据参数"() -> (w576:string)
      n294 = Format Into String(format string="#%s#" ("初始字符串"), w584) -> (resulting string=w591:string)  [unwired: 2 in, 1 out]
      n295 = Format Into String(format string="#%s#" ("初始字符串"), w583) -> (resulting string=w585:string)  [unwired: 2 in, 1 out]
      n296 = Concatenate Strings("where 测量模式 ='" ("condition"), w576, "' and 时间 between ", w591, "and" ("字符串"), w585) -> (w589:string)
      n297 = call "SQL查询.vi"("condition"=w589, "table输入"=w574, "database"="database1.mdb") -> ("error out"=w580:errorcluster, "data"=w582:string[][])  [unwired: 7 in]
      n298 = case shown="假" FALSE {
        tunnel: w582 -> [w593 w601]
        tunnel: [w593 w595] -> w581
        tunnel: w580 -> [w592 w594]
        tunnel: [w592 w594] -> w579
        frame False {
        }
        frame True {
          # "数字字符串精度转换保留"
          n299 = Index Array(array=w601, index (col)=3 ("禁用的索引 (列)")) -> (element=w602:string[])  [unwired: 1 in]
          n300 = for {
            tunnel: w602 -> [w605] mode=indexing
            tunnel: [w604] -> w597 mode=indexing
            n301 = Fract/Exp String To Number(string=w605) -> (number=w606:dbl)  [unwired: 3 in, 1 out]
            n302 = Number To Fractional String(number=w606, precision (6)=i16 2 ("精度(6)")) -> (F-format string=w604:string)  [unwired: 2 in]
          }
          n303 = Delete From Array(array=w601, length=1 ("长度"), index (col)=3 ("禁用的索引 (列)")) -> (array with subset deleted=w598:string[][])  [unwired: 1 in, 1 out]
          n304 = Insert Into Array(array=w598, index (col)=3 ("禁用的索引 (列)"), new element=w597) -> (w595:string[][])  [unwired: 1 in]
        }
      }
    }
  }
  "待发送数据" <- w3
  n305 = call <vilib>:"Clear Errors.vi"("error in (no error)"=w7) -> ("error out"=→"error out":errorcluster)  [unwired: 5 in, 1 out]
  n306 = Index Array(array=w3, index (row)=0 ("索引 (行)")) -> (element=→"待发送第一条数据":string[])  [unwired: 1 in]
